vi "ISO8601 DateString_subVI to Timestamp.vi"(9 "Strict ISO? (T)":bool=TRUE, 11 "ISO8601 Date String":string) -> (1 "valid?":bool, 2 "ISO Format":T1, 3 "Timestamp":timestamp)   [LabVIEW 2017]
uses:
  ISO8601 Date Formats.ctl
  <vilib>/Utility/miscctls.llb/LVDateTimeRec.ctl
  Timestamp to ISO8601 Day.vi
  isLeapYear (integer).vi
  <vilib>/regexp/Match Regular Expression.xnode
  DateTime.ISO8601.lvclass
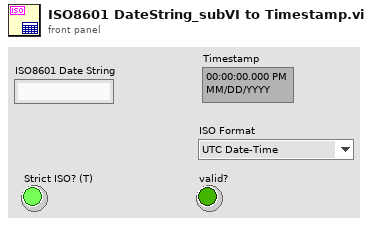
[diagram p1: front panel]
types:
  T1 = typedef "ISO8601 Date Formats.ctl" = enum16{"UTC Date-Time", "ISO Time", "Date", "Calendar Month", "Week", "Week-Day", "Month-Day", "Ordinal Date"}
  T2 = typedef "LVDateTimeRec.ctl" = cluster{"fractional second":dbl, "second":i32, "minute":i32, "hour":i32, "day of month":i32, "month":i32, "year":i32, "day of week":i32, "day of year":i32, "DST":i32}
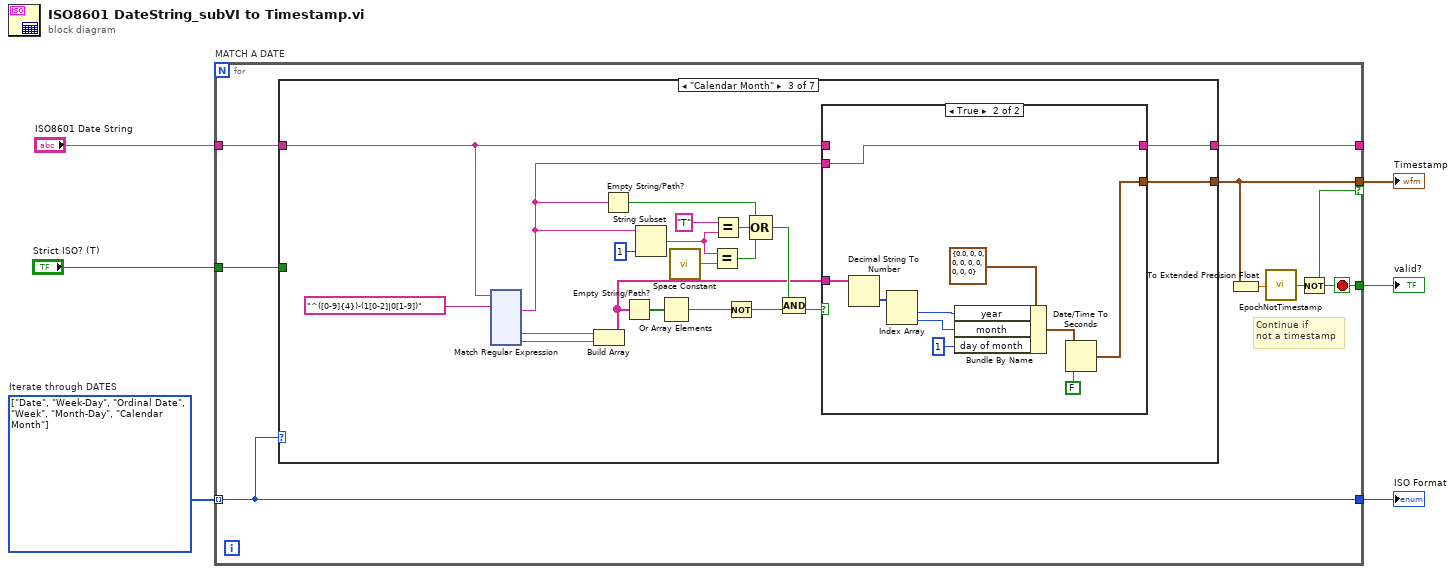
[diagram p0: block diagram]
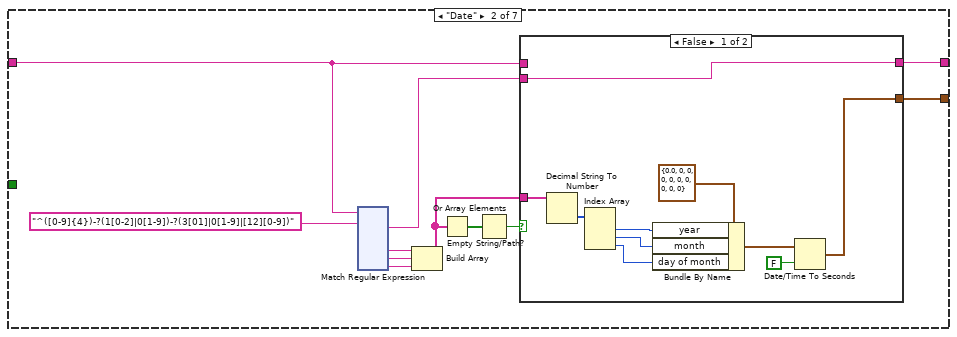
[diagram p3: hidden frame]
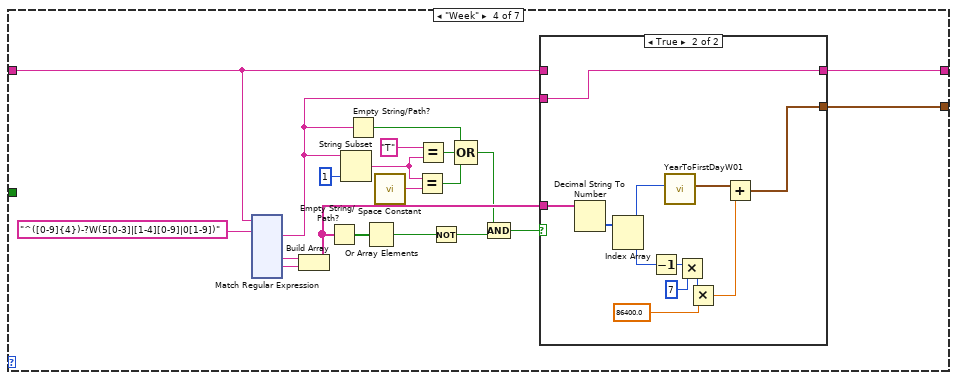
[diagram p6: hidden frame]
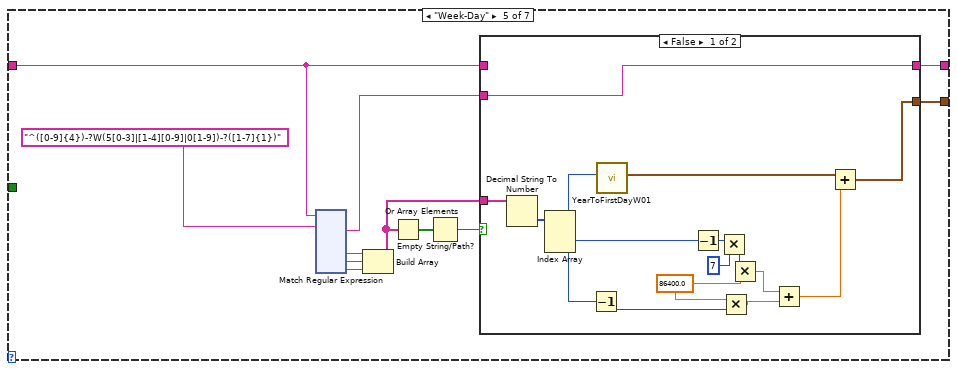
[diagram p8: hidden frame]
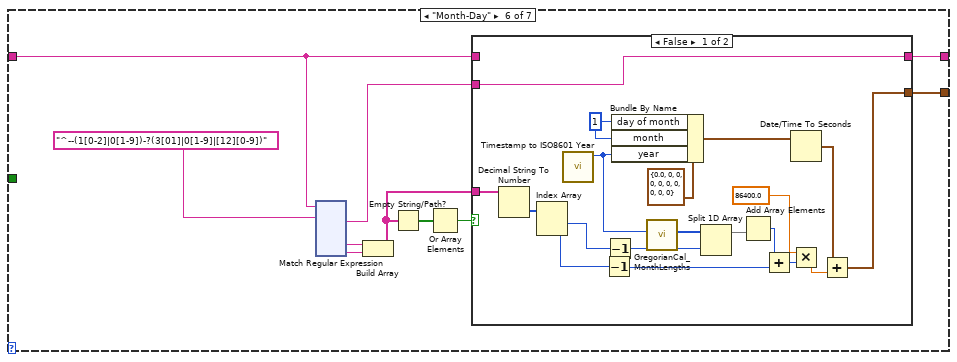
[diagram p10: hidden frame]
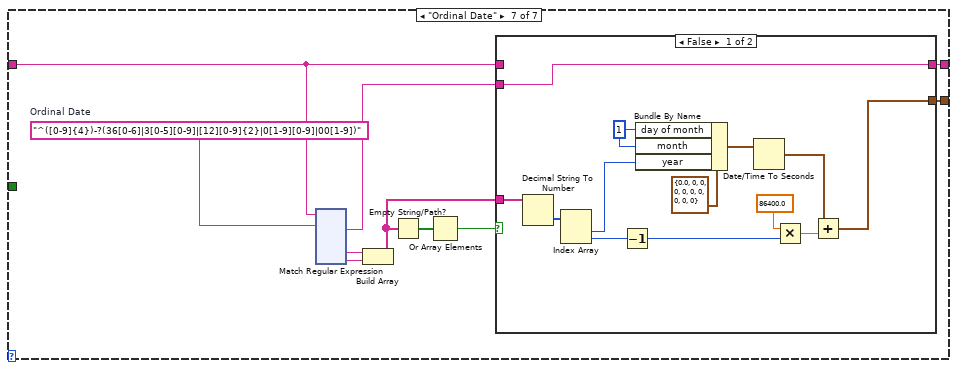
[diagram p12: hidden frame]
diagram:
  w1 = T1[] [enum."Date", enum."Week-Day", enum."Ordinal Date", enum."Week", enum."Month-Day", enum."Calendar Month"] items=["UTC Date-Time", "ISO Time", "Date", "Calendar Month", "Week", "Week-Day", "Month-Day", "Ordinal Date"]  # Iterate through DATES
  n1 = for "MATCH A DATE" {
    tunnel: "ISO8601 Date String" -> [w14]
    tunnel: [w7] -> w4
    tunnel: [w11] -> w5
    tunnel: w1 -> [w11] mode=indexing
    tunnel: "Strict ISO? (T)" -> [w10]
    tunnel: [w9] -> _
    tunnel: [w8] -> w3 if=w7
    stop <- w7 stop-if-true
    # "Continue if\nnot a timestamp"
    n2 = case shown="\"Calendar Month\"" w11 {
      tunnel: w14 -> [w15 w16 w159 w322 w464 w613 w763]
      tunnel: w10 -> [_ _ _ _ _ _ _]
      tunnel: [w15 w18 w177 w323 w465 w614 w765] -> w9
      tunnel: [_ w19 w178 w324 w467 w616 w766] -> w8
      frame Default {
        # "We process only DATES in this loop."
      }
      frame "Date" {
        n3 = xnode "Match Regular Expression"("input string"=w16, "regular expression"="^([0-9]{4})-?(1[0-2]|0[1-9])-?(3[01]|0[1-9]|[12][0-9])") -> ("after match"=w17:string, "submatch 1"=w26:string, "submatch 2"=w25:string, "submatch 3"=w24:string)  [unwired: 4 in, 4 out]
        n4 = Build Array(w26, w25, w24) -> (w20:string[])
        n5 = Empty String/Path?(string/path=w20) -> (empty?=w23:bool[])
        n6 = Or Array Elements(Boolean array=w23) -> (logical OR=w22:bool)
        n7 = case shown="False" w22 {
          tunnel: w20 -> [w156 _]
          tunnel: [w150 _] -> w19
          tunnel: [w149 w158] -> w18
          tunnel: w17 -> [w149 _]
          tunnel: w16 -> [_ w158]
          frame False {
            n8 = Decimal String To Number(string=w156) -> (number=w157:i32[])  [unwired: 2 in, 1 out]
            n9 = Index Array(array=w157) -> (element #1=w155:i32, element #2=w154:i32, element #3=w153:i32)  [unwired: 3 in]
            n10 = Bundle By Name(cluster=T2 {"fractional second"=0.0, "second"=0, "minute"=0, "hour"=0, "day of month"=0, "month"=0, "year"=0, "day of week"=0, "day of year"=0, "DST"=0} ("date time rec"), "year"=w155, "month"=w154, "day of month"=w153) -> (w152:T2)
            n11 = Date/Time To Seconds(1:FALSE ("is UTC (F)"), 2:w152) -> (0:w150:timestamp)
          }
          frame True {
          }
        }
      }
      frame "Calendar Month" {
        n12 = xnode "Match Regular Expression"("input string"=w159, "regular expression"="^([0-9]{4})-(1[0-2]|0[1-9])") -> ("after match"=w162:string, "submatch 1"=w163:string, "submatch 2"=w164:string)  [unwired: 4 in, 4 out]
        n13 = Build Array(w163, w164) -> (w161:string[])
        n14 = Empty String/Path?(string/path=w162) -> (empty?=w166:bool)
        n15 = Empty String/Path?(string/path=w161) -> (empty?=w165:bool[])
        n16 = String Subset(string=w162, length (rest)=1 ("length (rest)")) -> (substring=w170:string)  [unwired: 1 in]
        n17 = Or Array Elements(Boolean array=w165) -> (logical OR=w174:bool)
        n18 = call <vilib>:"Space Constant.vi"() -> ("String"=w172:string)
        n19 = Equal?(x=w170, y=w172) -> (x = y?=w171:bool)
        n20 = Equal?(x="T", y=w170) -> (x = y?=w169:bool)
        n21 = Not(x=w174) -> (.not. x?=w175:bool)
        n22 = Compound Arithmetic op=OR(w166, w169, w171) -> (w173:bool)
        n23 = Compound Arithmetic op=AND(w173, w175) -> (w160:bool)
        n24 = case shown="True" w160 {
          tunnel: w161 -> [_ w306]
          tunnel: [_ w301] -> w178
          tunnel: w159 -> [w299 _]
          tunnel: [w299 w300] -> w177
          tunnel: w162 -> [_ w300]
          frame False {
          }
          frame True {
            n25 = Decimal String To Number(string=w306) -> (number=w308:i32[])  [unwired: 2 in, 1 out]
            n26 = Index Array(array=w308) -> (element #1=w305:i32, element #2=w304:i32)  [unwired: 2 in]
            n27 = Bundle By Name(cluster=T2 {"fractional second"=0.0, "second"=0, "minute"=0, "hour"=0, "day of month"=0, "month"=0, "year"=0, "day of week"=0, "day of year"=0, "DST"=0} ("date time rec"), "year"=w305, "month"=w304, "day of month"=1) -> (w303:T2)
            n28 = Date/Time To Seconds(1:FALSE ("is UTC (F)"), 2:w303) -> (0:w301:timestamp)
          }
        }
      }
      frame "Week" {
        n29 = xnode "Match Regular Expression"("input string"=w322, "regular expression"="^([0-9]{4})-?W(5[0-3]|[1-4][0-9]|0[1-9])") -> ("after match"=w320:string, "submatch 1"=w329:string, "submatch 2"=w328:string)  [unwired: 4 in, 5 out]
        n30 = Build Array(w329, w328) -> (w325:string[])
        n31 = Empty String/Path?(string/path=w325) -> (empty?=w327:bool[])
        n32 = String Subset(string=w320, length (rest)=1 ("length (rest)")) -> (substring=w316:string)  [unwired: 1 in]
        n33 = Empty String/Path?(string/path=w320) -> (empty?=w321:bool)
        n34 = Or Array Elements(Boolean array=w327) -> (logical OR=w312:bool)
        n35 = call <vilib>:"Space Constant.vi"() -> ("String"=w314:string)
        n36 = Equal?(x=w316, y=w314) -> (x = y?=w315:bool)
        n37 = Equal?(x="T", y=w316) -> (x = y?=w317:bool)
        n38 = Not(x=w312) -> (.not. x?=w311:bool)
        n39 = Compound Arithmetic op=OR(w321, w317, w315) -> (w313:bool)
        n40 = Compound Arithmetic op=AND(w313, w311) -> (w310:bool)
        n41 = case shown="True" w310 {
          tunnel: w325 -> [_ w462]
          tunnel: [_ w453] -> w324
          tunnel: [w451 w452] -> w323
          tunnel: w320 -> [_ w452]
          tunnel: w322 -> [w451 _]
          frame False {
          }
          frame True {
            n42 = Decimal String To Number(string=w462) -> (number=w463:i32[])  [unwired: 2 in, 1 out]
            n43 = Index Array(array=w463) -> (element #1=w461:i32, element #2=w460:i32)  [unwired: 2 in]
            n44 = Decrement(x=w460) -> (x-1=w459:i32)
            n45 = call "YearToFirstDayW01.vi"("year"=w461) -> ("First Day of W01"=w455:timestamp)  [unwired: 10 in]
            n46 = Multiply(x=w459, y=7) -> (x*y=w458:i32)
            n47 = Multiply(x=w458, y=86400.0) -> (x*y=w454:dbl)
            n48 = Add(x=w455, y=w454) -> (x+y=w453:timestamp)
          }
        }
      }
      frame "Week-Day" {
        n49 = xnode "Match Regular Expression"("input string"=w464, "regular expression"="^([0-9]{4})-?W(5[0-3]|[1-4][0-9]|0[1-9])-?([1-7]{1})") -> ("after match"=w466:string, "submatch 1"=w474:string, "submatch 2"=w473:string, "submatch 3"=w469:string)  [unwired: 4 in, 4 out]
        n50 = Build Array(w474, w473, w469) -> (w470:string[])
        n51 = Empty String/Path?(string/path=w470) -> (empty?=w472:bool[])
        n52 = Or Array Elements(Boolean array=w472) -> (logical OR=w471:bool)
        n53 = case shown="False" w471 {
          tunnel: w470 -> [w610 _]
          tunnel: [w597 _] -> w467
          tunnel: [w596 w612] -> w465
          tunnel: w466 -> [w596 _]
          tunnel: w464 -> [_ w612]
          frame False {
            w600 = 86400.0
            n54 = Decimal String To Number(string=w610) -> (number=w611:i32[])  [unwired: 2 in, 1 out]
            n55 = Index Array(array=w611) -> (element #1=w609:i32, element #2=w608:i32, element #3=w601:i32)  [unwired: 3 in]
            n56 = Decrement(x=w601) -> (x-1=w599:i32)
            n57 = call "YearToFirstDayW01.vi"("year"=w609) -> ("First Day of W01"=w604:timestamp)  [unwired: 10 in]
            n58 = Decrement(x=w608) -> (x-1=w607:i32)
            n59 = Multiply(x=w607, y=7) -> (x*y=w606:i32)
            n60 = Multiply(x=w600, y=w599) -> (x*y=w598:dbl)
            n61 = Multiply(x=w606, y=w600) -> (x*y=w603:dbl)
            n62 = Add(x=w603, y=w598) -> (x+y=w602:dbl)
            n63 = Add(x=w604, y=w602) -> (x+y=w597:timestamp)
          }
          frame True {
          }
        }
      }
      frame "Month-Day" {
        n64 = xnode "Match Regular Expression"("input string"=w613, "regular expression"="^--(1[0-2]|0[1-9])-?(3[01]|0[1-9]|[12][0-9])") -> ("after match"=w615:string, "submatch 1"=w622:string, "submatch 2"=w621:string)  [unwired: 4 in, 4 out]
        n65 = Build Array(w622, w621) -> (w618:string[])
        n66 = Empty String/Path?(string/path=w618) -> (empty?=w620:bool[])
        n67 = Or Array Elements(Boolean array=w620) -> (logical OR=w619:bool)
        n68 = case shown="False" w619 {
          tunnel: w618 -> [w760 _]
          tunnel: [w744 _] -> w616
          tunnel: w615 -> [w743 _]
          tunnel: [w743 w762] -> w614
          tunnel: w613 -> [_ w762]
          frame False {
            w756 = 1 ("day of month")
            n69 = Decimal String To Number(string=w760) -> (number=w761:i32[])  [unwired: 2 in, 1 out]
            n70 = Index Array(array=w761) -> (element #1=w751:i32, element #2=w759:i32)  [unwired: 2 in]
            n71 = call "Timestamp to ISO8601 Year.vi"() -> ("year"=w753:i32)  [unwired: 10 in, 1 out]
            n72 = Decrement(x=w759) -> (x-1=w747:i32)
            n73 = Decrement(x=w751) -> (x-1=w750:i32)
            n74 = Bundle By Name(cluster=T2 {"fractional second"=0.0, "second"=0, "minute"=0, "hour"=0, "day of month"=0, "month"=0, "year"=0, "day of week"=0, "day of year"=0, "DST"=0} ("date time rec"), "day of month"=w756, "month"=w756, "year"=w753) -> (w757:T2)
            n75 = call "GregorianCal_MonthLengths.vi"("Year (0: this year)"=w753) -> ("Month Lengths"=w752:i32[])  [unwired: 10 in]
            n76 = Split 1D Array(array=w752, index=w750) -> (first subarray=w749:i32[])  [unwired: 1 out]
            n77 = Add Array Elements(numeric array=w749) -> (sum=w748:i32)
            n78 = Add(x=w748, y=w747) -> (x+y=w746:i32)
            n79 = Date/Time To Seconds(2:w757) -> (0:w754:timestamp)  [unwired: 1 in]
            n80 = Multiply(x=86400.0, y=w746) -> (x*y=w745:dbl)
            n81 = Add(x=w754, y=w745) -> (x+y=w744:timestamp)
          }
          frame True {
          }
        }
      }
      frame "Ordinal Date" {
        w767 = "^([0-9]{4})-?(36[0-6]|3[0-5][0-9]|[12][0-9]{2}|0[1-9][0-9]|00[1-9])"  # Ordinal Date
        n82 = xnode "Match Regular Expression"("input string"=w763, "regular expression"=w767) -> ("after match"=w764:string, "submatch 1"=w772:string, "submatch 2"=w771:string)  [unwired: 4 in, 4 out]
        n83 = Build Array(w772, w771) -> (w768:string[])
        n84 = Empty String/Path?(string/path=w768) -> (empty?=w770:bool[])
        n85 = Or Array Elements(Boolean array=w770) -> (logical OR=w769:bool)
        n86 = case shown="False" w769 {
          tunnel: w768 -> [w904 _]
          tunnel: [w893 _] -> w766
          tunnel: [w894 w906] -> w765
          tunnel: w764 -> [w894 _]
          tunnel: w763 -> [_ w906]
          frame False {
            w900 = 1 ("day of month")
            n87 = Decimal String To Number(string=w904) -> (number=w905:i32[])  [unwired: 2 in, 1 out]
            n88 = Index Array(array=w905) -> (element #1=w897:i32, element #2=w903:i32)  [unwired: 2 in]
            n89 = Decrement(x=w903) -> (x-1=w896:i32)
            n90 = Bundle By Name(cluster=T2 {"fractional second"=0.0, "second"=0, "minute"=0, "hour"=0, "day of month"=0, "month"=0, "year"=0, "day of week"=0, "day of year"=0, "DST"=0} ("date time rec"), "day of month"=w900, "month"=w900, "year"=w897) -> (w901:T2)
            n91 = Date/Time To Seconds(2:w901) -> (0:w895:timestamp)  [unwired: 1 in]
            n92 = Multiply(x=86400.0, y=w896) -> (x*y=w898:dbl)
            n93 = Add(x=w895, y=w898) -> (x+y=w893:timestamp)
          }
          frame True {
          }
        }
      }
    }
    n94 = To Extended Precision Float(1:w8) -> (0:w13:ext)
    n95 = call "EpochNotTimestamp.vi"("Epoch Time"=w13) -> ("Not a Timestamp?"=w12:bool)  [unwired: 8 in]
    n96 = Not(x=w12) -> (.not. x?=w7:bool)
  }
  "ISO Format" <- w5
  "valid?" <- w4
  "Timestamp" <- w3
